vi "Digital Filter.vi"(10 "Tics to Filter":fxp<+,11,11>, 11 "Input Signal":bool) -> (3 "Output Filtered Signal":bool)   [LabVIEW 2013]
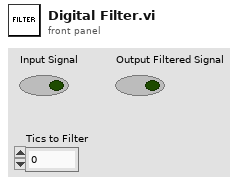
[diagram p1: front panel]
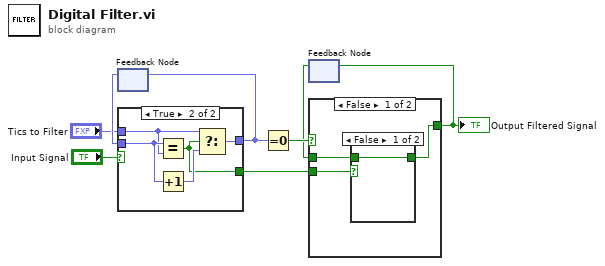
[diagram p0: block diagram]
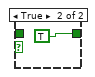
[diagram p2: hidden frame]
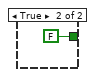
[diagram p3: hidden frame]
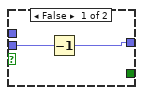
[diagram p4: hidden frame]
diagram:
  n1 = feedback #1() -> (w8:fxp<+,11,11>)  [unwired: 1 in]
  n2 = case shown="True" "Input Signal" {
    tunnel: [w9 w12] -> w5
    tunnel: w8 -> [w10 w15]
    tunnel: "Tics to Filter" -> [_ w13]
    tunnel: [_ w11] -> w1
    frame False {
      n3 = Decrement(x=w10) -> (x-1=w9:fxp<+,11,11>)
    }
    frame True {
      n4 = Equal?(x=w15, y=w13) -> (x = y?=w11:bool)
      n5 = Increment(x=w15) -> (x+1=w14:fxp<+,11,11>)
      n6 = Select(t=w13, s=w11, f=w14) -> (s? t:f=w12:fxp<+,11,11>)
    }
  }
  n7 = feedback-in #1(w5) -> ()
  n8 = Equal To 0?(x=w5) -> (x = 0?=w4:bool)
  n9 = feedback #2() -> (w3:bool)  [unwired: 1 in]
  n10 = case shown="False" w4 {
    tunnel: w3 -> [w16 _]
    tunnel: [w17 FALSE] -> w2
    tunnel: w1 -> [w18 _]
    frame False {
      n11 = case shown="False" w18 {
        tunnel: [w19 TRUE] -> w17
        tunnel: w16 -> [w19 _]
        frame False {
        }
        frame True {
        }
      }
    }
    frame True {
    }
  }
  "Output Filtered Signal" <- w2
  n12 = feedback-in #2(w2) -> ()
